vi "Initialize.vi"(8 "error in":errorcluster, 10 "parameters":variant, 11 "node in":refnum<class "Temperature.lvclass">) -> (0 "error out":errorcluster, 2 "summary":T2[](array[typedef]), 3 "data value reference":T1)   [LabVIEW 2015, in "Temperature.lvclass"]
doc: "Initializes the data of a node to its default state.\nThe object is not created inside of this VI, because it is created from a File depending on user selection."
uses:
  Temperature.lvclass
  <vilib>/NI/Configuration Framework/Node/Summary.ctl
  <vilib>/NI/Configuration Framework/Node/NodeRef.ctl
  <vilib>/NI/Configuration Framework/Node/NISE_CEF_Node.lvclass
  cRIO Repo/ChannelData.ctl
  Channel/Channel.lvclass/Channel.ctl
  Channel/Write Channel info.vi
  Channel/Channel.lvclass
  cRIO Repo/cRIORepo.lvclass
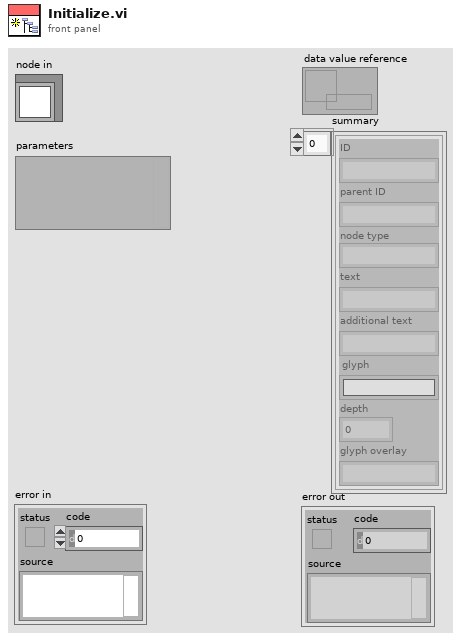
[diagram p1: front panel]
types:
  T1 = typedef "NISE_CEF_Node.lvclass/NodeRef.ctl" = refnum<data-value>
  T2 = typedef "NISE_CEF_Node.lvclass/Summary.ctl" = cluster{"ID":string, "parent ID":string, "node type":string, "text":string, "additional text":string, "glyph":string, "depth":i32, "glyph overlay":string}
  T3 = typedef "cRIORepo.lvclass/ChannelData.ctl" = cluster{"channel group":string, "channel name":string, "IO ":string, "sensor ID":string, "description":string, "system":string, "channel type":string}
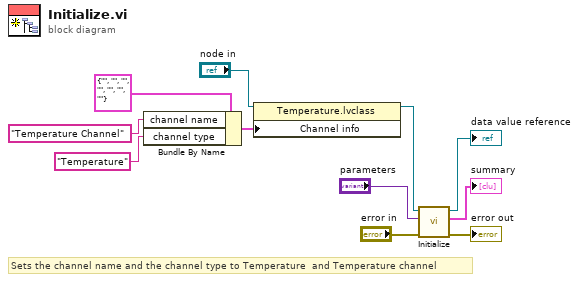
[diagram p0: block diagram]
diagram:
  # "Sets the channel name and the channel type to Temperature  and Temperature channel"
  n1 = Bundle By Name(cluster=T3 {"channel group"="", "channel name"="", "IO "="", "sensor ID"="", "description"="", "system"="", "channel type"=""} ("channel info"), "channel name"="Temperature Channel" ("channel Name"), "channel type"="Temperature" ("channelType")) -> (w5:T3)
  n2 = property class="Temperature.lvclass"(reference="node in", "Channel info"=w5) -> (reference out=w1:refnum<class "Temperature.lvclass">)  [unwired: 1 in, 1 out]
  n3 = call-parent "Initialize.vi"("error in"="error in", "parameters"="parameters", "node in"=w1) -> ("error out"=→"error out":errorcluster, "summary"=→"summary":T2[], "data value reference"=→"data value reference":T1)  [unwired: 6 in]
